vi "Shift Rows3.vi"(7 "Nb":i32=4, 8 "error in":errorcluster, 10 "State In":u16[][](array[numeric])=[[255, 97, 23, 96], [160, 160, 73, 200], [205, 24, 172, 154], [50, 93, 135, 180]]) -> (0 "error out":errorcluster, 2 "State Out":u16[][](array[numeric]))   [LabVIEW 2016, in "数据传输系统-04.lvlib"]
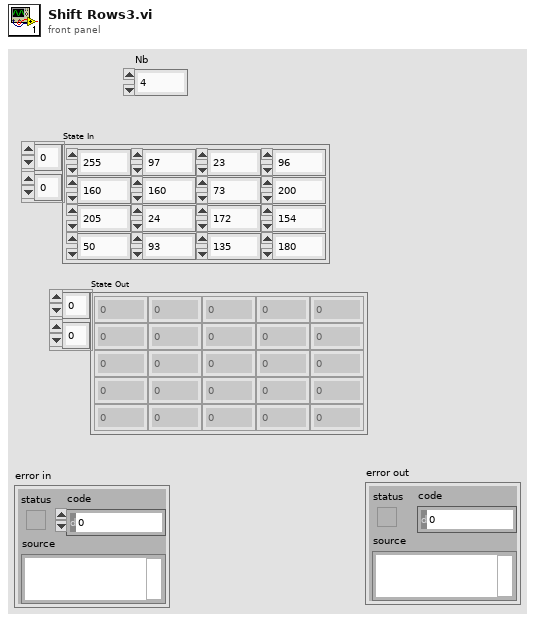
[diagram p1: front panel]
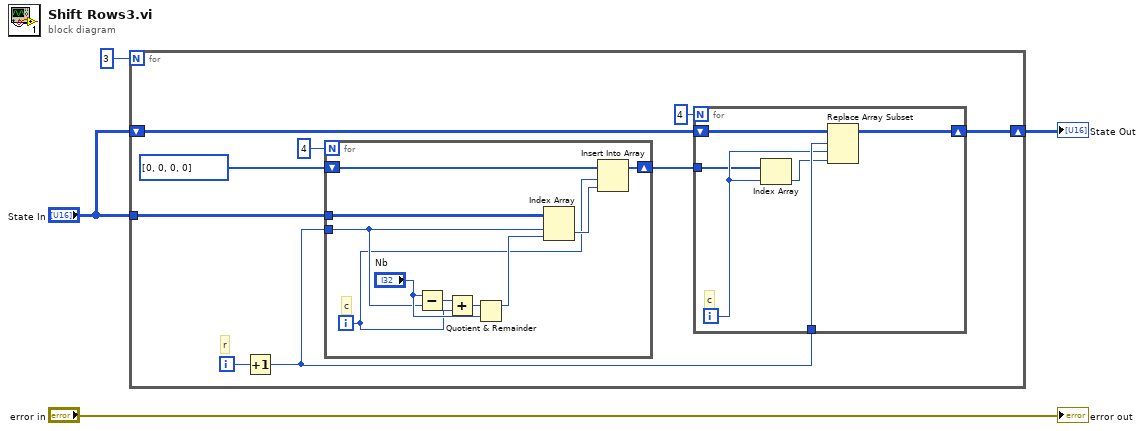
[diagram p0: block diagram]
diagram:
  n1 = for {
    N: 3 -> [_]
    tunnel: "State In" -> [w13]
    shift-right: [w9] -> w2
    shift-left: "State In" -> [w10]
    i -> [w12]
    # "r"
    n2 = Increment(x=w12) -> (x+1=w11:i32)
    n3 = for {
      N: 4 -> [_]
      tunnel: w13 -> [w29]
      tunnel: w11 -> [w23]
      shift-right: [w27] -> w7
      shift-left: i32[] [0, 0, 0, 0] ("t[c]") -> [w28]
      i -> [w21]
      # "c"
      n4 = Subtract(x="Nb", y=w23) -> (x-y=w22:i32)
      n5 = Add(x=w22, y=w21) -> (x+y=w20:i32)
      n6 = Quotient & Remainder(x=w20, y="Nb") -> (x-y*floor(x/y)=w26:i32)  [unwired: 1 out]
      n7 = Index Array(array=w29, index (row)=w23, index (col)=w26) -> (element=w25:u16)
      n8 = Insert Into Array(array=w28, index=w21, new element=w25) -> (w27:i32[])
    }
    n9 = for {
      N: 4 -> [_]
      tunnel: w11 -> [w19]
      shift-right: [w15] -> w9
      shift-left: w10 -> [w16]
      tunnel: w7 -> [w14]
      i -> [w18]
      # "c"
      n10 = Index Array(array=w14, index=w18) -> (element=w17:i32)
      n11 = Replace Array Subset(array=w16, new element=w17, index (row)=w19, index (col)=w18) -> (w15:u16[][])
    }
  }
  "State Out" <- w2
  "error out" <- "error in"
